vi "GetSampleName.vi"(4 "Transducer":T1, 5 "Sanmple Name":string) -> (0 "Canceled":bool, 1 "Transducer":T1, 2 "Name":string)   [LabVIEW 2022 SP3]
uses:
  Controls/HF_XDCRs.ctl
panel:
  in  "Cancel":bool
  in  "OK":bool
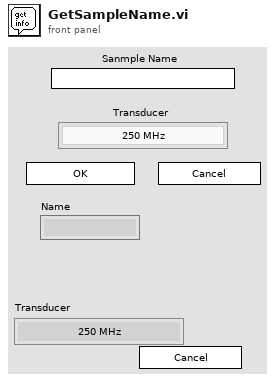
[diagram p1: front panel]
types:
  T1 = typedef "HF_XDCRs.ctl" = enum16{"250 MHz", "500 MHz"}
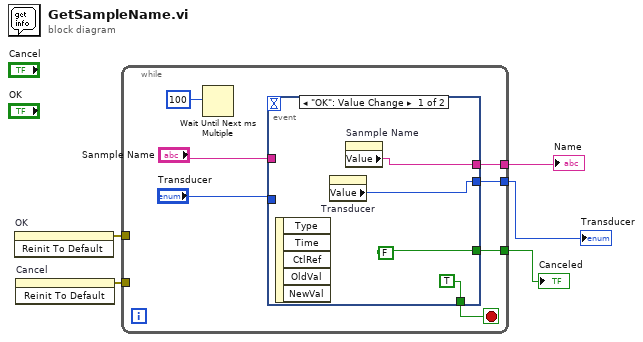
[diagram p0: block diagram]
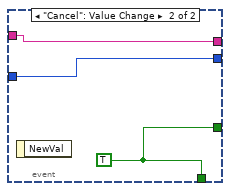
[diagram p2: hidden frame]
diagram:
  n1 = invoke on="OK" class="Bool" method="Reinit To Default"() -> (error out=w5:errorcluster)  [unwired: 3 in, 2 out]
  n2 = invoke on="Cancel" class="Bool" method="Reinit To Default"() -> (error out=w4:errorcluster)  [unwired: 3 in, 2 out]
  n3 = while {
    tunnel: w5 -> [_]
    tunnel: w4 -> [_]
    tunnel: [w10] -> w3
    tunnel: [w7] -> w2
    tunnel: [w6] -> w1
    stop <- w11 stop-if-true
    n4 = Wait Until Next ms Multiple(millisecond multiple=100) -> ()  [unwired: 1 out]
    n5 = event shown="[0] \"OK\": Value Change" {
      selector: _ -> [_ _]
      dyn-events: _ -> [_ _]
      timeout: _ -> [_ _]
      tunnel: [TRUE w17] -> w11
      tunnel: [w14 w19] -> w6
      tunnel: [w13 w18] -> w7
      tunnel: [FALSE w17] -> w10
      tunnel: "Sanmple Name" -> [_ w19]
      tunnel: "Transducer" -> [_ w18]
      event "OK": Value Change {
        n6 = event-data() -> ()  [unwired: 6 out]
        n7 = property on="Transducer" class="Enum (strict)"() -> ("Value"=w13:T1)  [unwired: 2 in, 2 out]
        n8 = property on="Sanmple Name" class="Str"() -> ("Value"=w14:string)  [unwired: 2 in, 2 out]
      }
      event "Cancel": Value Change {
        w17 = TRUE
        n9 = event-data() -> ()  [unwired: 2 out]
      }
    }
  }
  "Name" <- w1
  "Transducer" <- w2
  "Canceled" <- w3
